vi "Scale_ADC Data.vi"(8 "error in (no error)":errorcluster, 11 "DAQ_Device in":refnum<class "DAQ_Device.lvclass">) -> (0 "error out":errorcluster, 3 "DAQ_Device out":refnum<class "DAQ_Device.lvclass">)   [LabVIEW 2023, in "DAQ_Device.lvclass"]
uses:
  DAQ_Device.lvclass
  DAQ Device_ChannelConfiguration.ctl
panel:
  in  "ADC/Register Value":u32
  in  "input cluster":T1={"Name"="", "InputType"=enum."Voltage (+/- 10V)", "UL"=0.0, "LL"=0.0, "GAIN"=0.0, "OFFSET"=0.0, "FACTOR"=0.0}
  out "output variable":dbl
  out "InRange?":bool
  out "Value":dbl
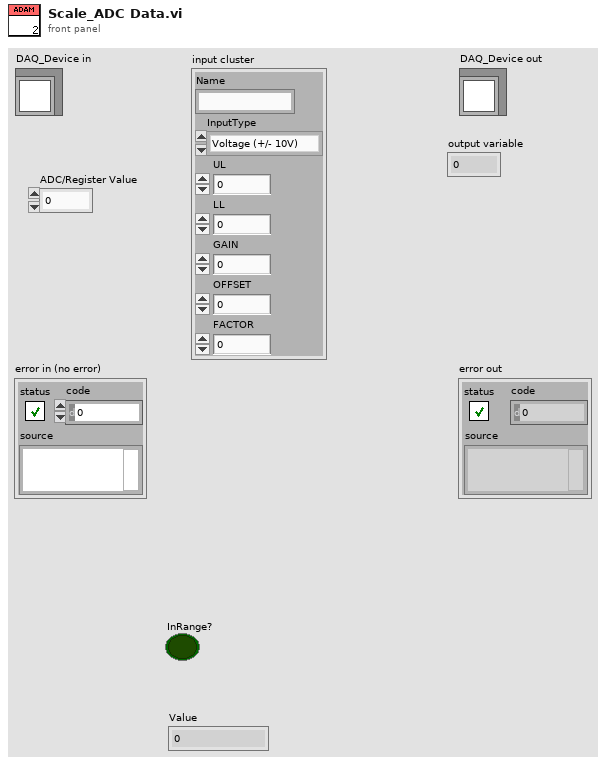
[diagram p1: front panel]
types:
  T1 = typedef "DAQ Device_ChannelConfiguration.ctl" = cluster{"Name":string, "InputType":enum16{"MB Register", "Current (4-20 mA)", "Current (0-20 mA)", "Voltage (+/- 10V)"}, "UL":dbl, "LL":dbl, "GAIN":dbl, "OFFSET":dbl, "FACTOR":dbl}
  T2 = enum16{"MB Register", "Current (4-20 mA)", "Current (0-20 mA)", "Voltage (+/- 10V)"}
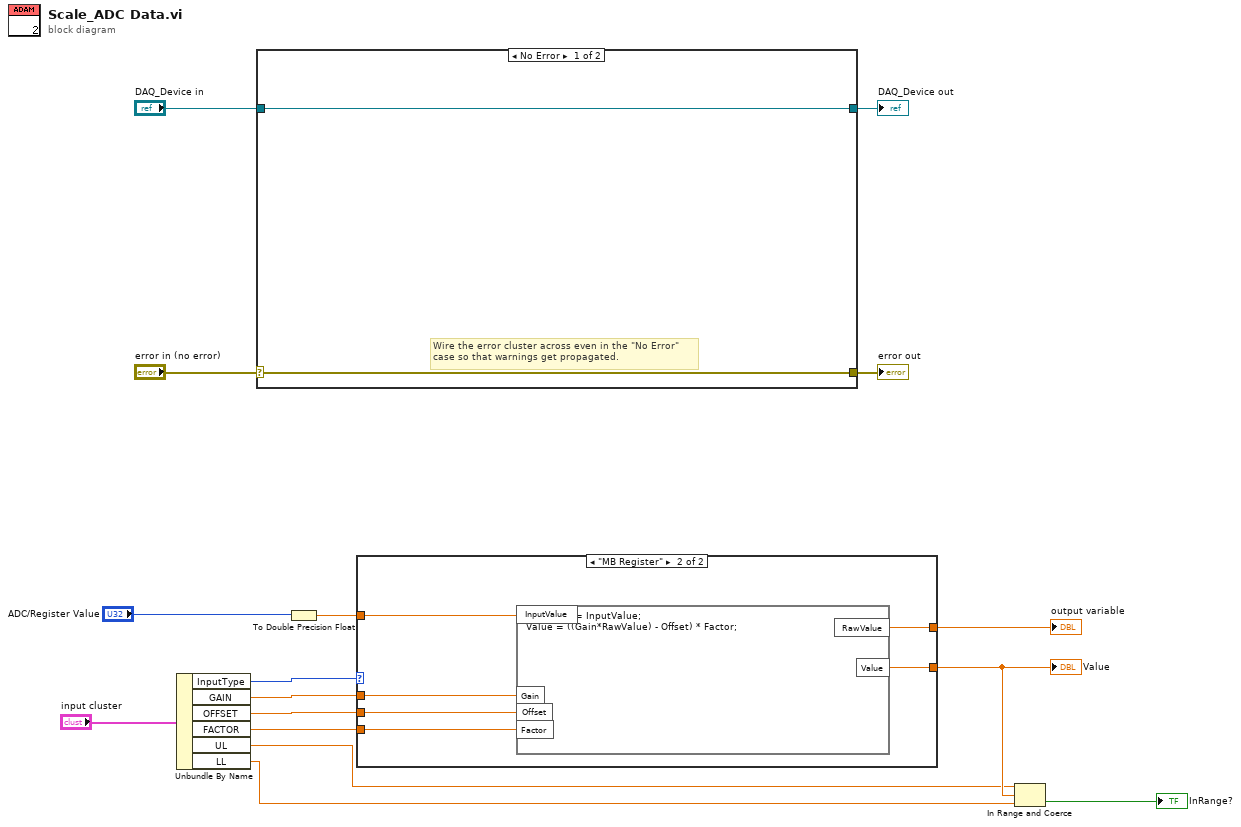
[diagram p0: block diagram]
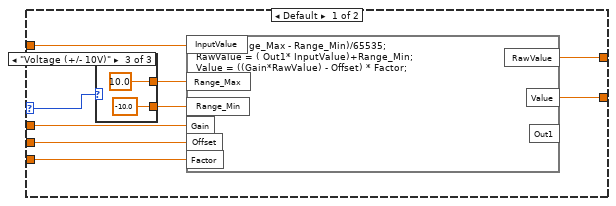
[diagram p2: hidden frame]
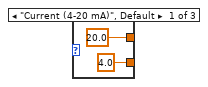
[diagram p3: hidden frame]
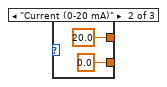
[diagram p4: hidden frame]
diagram:
  n1 = Unbundle By Name("input cluster") -> ("InputType"=w4:T2, "GAIN"=w12:dbl, "OFFSET"=w11:dbl, "FACTOR"=w10:dbl, "UL"=w6:dbl, "LL"=w7:dbl)
  n2 = case shown="No Error" "error in (no error)" {
    selector: "error in (no error)" -> [w17 w20]
    tunnel: [w17 w20] -> w15
    tunnel: [w18 w19] -> w13
    tunnel: "DAQ_Device in" -> [w18 w19]
    frame No Error {
      # "Wire the error cluster across even in the \"No Error\"\ncase so that warnings get propagated."
    }
    frame Error {
    }
  }
  "error out" <- w15
  "DAQ_Device out" <- w13
  n3 = To Double Precision Float(number="ADC/Register Value") -> (double precision float=w1:dbl)
  n4 = case shown="\"MB Register\"" w4 {
    selector: w4 -> [w22 _]
    tunnel: w12 -> [w29 w41]
    tunnel: w11 -> [w28 w40]
    tunnel: w10 -> [w27 w39]
    tunnel: [w24 w38] -> w9
    tunnel: [w23 w37] -> w8
    tunnel: w1 -> [w21 w36]
    frame Default {
      n5 = case shown="\"Voltage (+/- 10V)\"" w22 {
        tunnel: [4.0 ("y") 0.0 ("y") -10.0 ("y")] -> w25
        tunnel: [20.0 ("y") 20.0 ("y") 10.0 ("y")] -> w26
        frame "Current (4-20 mA)", Default {
        }
        frame "Current (0-20 mA)" {
        }
        frame "Voltage (+/- 10V)" {
        }
      }
      n6 = formula code="Out1=(Range_Max - Range_Min)/65535;\nRawValue = ( Out1* InputValue)+Range_Min;\nValue = ((Gain*RawValue) - Offset) * Factor;"("Gain"=w29, "Offset"=w28, "Factor"=w27, "Range_Min"=w25, "Range_Max"=w26, "InputValue"=w21) -> ("Value"=w23:dbl, "RawValue"=w24:dbl)  [unwired: 1 out]
    }
    frame "MB Register" {
      n7 = formula code="RawValue = InputValue;\nValue = ((Gain*RawValue) - Offset) * Factor;"("Gain"=w41, "Offset"=w40, "Factor"=w39, "InputValue"=w36) -> ("Value"=w37:dbl, "RawValue"=w38:dbl)
    }
  }
  "Value" <- w8
  "output variable" <- w9
  n8 = In Range and Coerce(upper limit=w6, x=w8, lower limit=w7) -> (In Range?=→"InRange?":bool)  [unwired: 1 out]
